vi "CMD_Global.vi"() -> ()   [LabVIEW 2017]
uses:
  _SOURCE2018_Master/_SHARE ALL/RoboRio Share All/SRX Share All/TypeDefs SRX/Cluster_SRX_Mode and Value.ctl
  _SOURCE2018_Master/System Drivers/Phoenix-LabVIEW/Motor Controller/Controls/CTRE_Phoenix_MotorControl_ControlMode.ctl
panel:
  in  "CMD_LeftMotor":T1 {"Mode" items=["PercentOutput"=0, "Position"=1, "Velocity"=2, "Current"=3, "Follower"=5, "MotionProfile"=6, "MotionMagic"=7, "MotionMagicArc"=8, "MotionProfileArc"=10, "Disabled"=15]}
  in  "CMD_RightMotor":T1 {"Mode" items=["PercentOutput"=0, "Position"=1, "Velocity"=2, "Current"=3, "Follower"=5, "MotionProfile"=6, "MotionMagic"=7, "MotionMagicArc"=8, "MotionProfileArc"=10, "Disabled"=15]}
  # "The Names of the Data items in the Global Variable MUST describe who the Single Writer is\nNaming Convention of all Data Items is:   \nCMD_Data Name\nExamples:\nCMD_Drive Data"
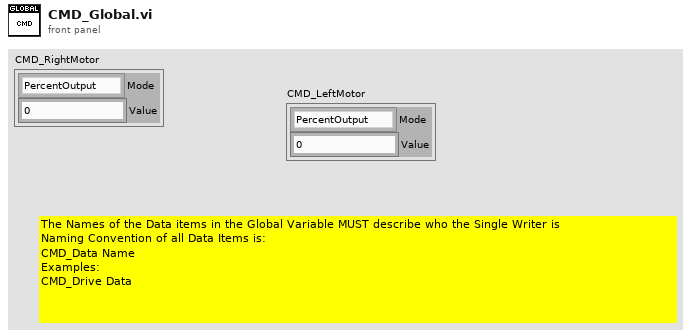
[diagram p1: front panel]
types:
  T1 = typedef "Cluster_SRX_Mode and Value.ctl" = cluster{"Mode":T2, "Value":dbl}
  T2 = typedef "CTRE_Phoenix_MotorControl_ControlMode.ctl" = u16
diagram:
